vi "Piece_file_Copy.vi"(1 "File Start String":string, 2 "Start to copy file at:":i32, 3 "Source File":path, 4 "Target File":path) -> ()   [LabVIEW 2010]
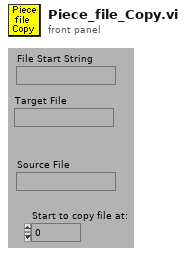
[diagram p1: front panel]
types:
  T1 = enum16{"read/write", "read-only", "write-only", "write-only (truncate)"}
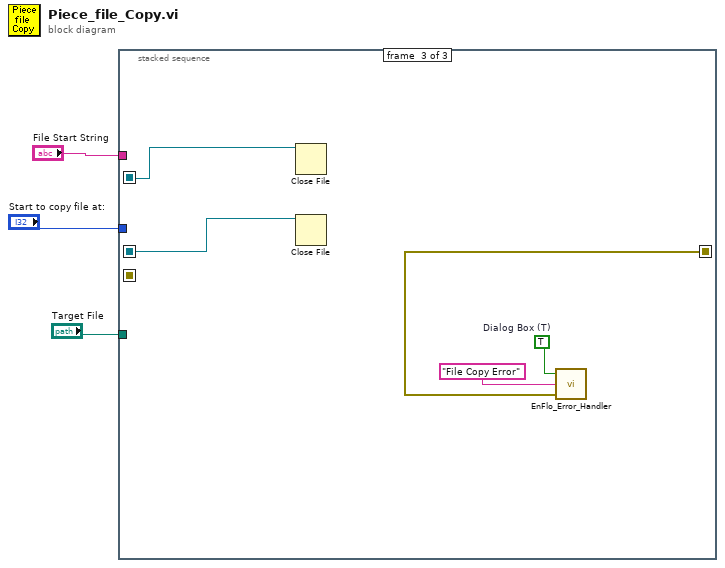
[diagram p0: block diagram]
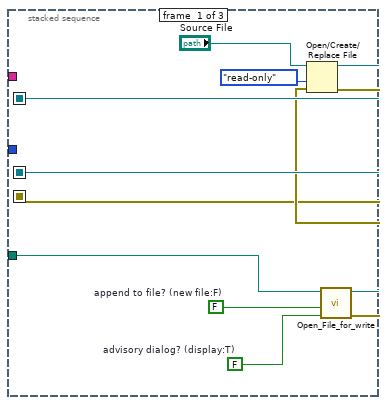
[diagram p2: hidden frame]
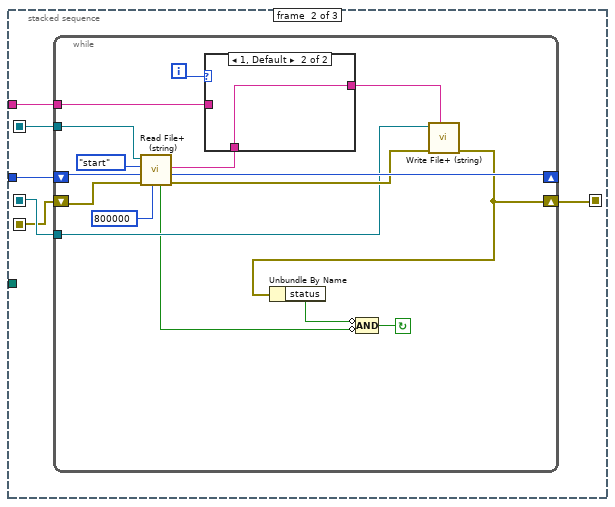
[diagram p3: hidden frame]
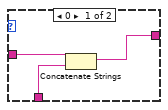
[diagram p4: hidden frame]
diagram:
  n1 = stacked-sequence {
    seq-local: [w9 _ _] -> [_ w18 w43]
    seq-local: [w11 _ _] -> [_ w16 w42]
    seq-local: [w7 _ _] -> [_ w15 _]
    seq-local: [_ w14 _] -> [_ _ w40]
    tunnel: "File Start String" -> [_ w17 _]
    tunnel: "Target File" -> [w6 _ _]
    tunnel: "Start to copy file at:" -> [_ w13 _]
    frame #0 {
      w4 = FALSE  # advisory dialog? (display:T)
      w12 = FALSE  # append to file? (new file:F)
      n2 = call "Open_File_for_write.vi"("advisory dialog? (display:T)"=w4, "append to file? (new file:F)"=w12, "file path"=w6) -> ("error out"=w8:errorcluster, "refnum"=w11:refnum<file>)  [unwired: 7 out]
      n3 = Open/Create/Replace File(file path (use dialog)="Source File", error in=w8, access (0:read/write)=T1."read-only" ("open mode (0)")) -> (refnum out=w9:refnum<file>, error out=w7:errorcluster)  [unwired: 4 out]
    }
    frame #1 {
      n4 = while {
        shift-left: w15 -> [w24]
        shift-right: [w23] -> w14
        tunnel: w16 -> [w26]
        tunnel: w17 -> [w29]
        shift-left: w13 -> [w19]
        shift-right: [w31] -> _
        tunnel: w18 -> [w32]
        i -> [w28]
        stop <- w20 continue-if-true
        n5 = call <vilib>:"Read File+ (string).vi"("count"=800000, "error in (no error)"=w24, "pos offset (bytes:0)"=w19, "pos mode (rel. to current:2)"=enum16{"start", "end", "current"}."start", "refnum"=w32) -> ("error out"=w27:errorcluster, "mark after read (bytes)"=w31:i32, "string"=w30:string, "EOF?"=w21:bool)  [unwired: 3 out]
        n6 = case shown="1, Default" w28 {
          tunnel: w30 -> [w37 w38]
          tunnel: w29 -> [w36 _]
          tunnel: [w35 w38] -> w25
          frame 0 {
            n7 = Concatenate Strings(w36, w37) -> (w35:string)
          }
          frame 1, Default {
          }
        }
        n8 = call <vilib>:"Write File+ (string).vi"("string"=w25, "error in (no error)"=w27, "refnum"=w26) -> ("error out"=w23:errorcluster)  [unwired: 2 in, 4 out]
        n9 = Unbundle By Name(w23) -> ("status"=w22:bool)
        n10 = Compound Arithmetic op=AND(invert w22, invert w21) -> (w20:bool)
      }
    }
    frame #2 {
      w41 = TRUE  # Dialog Box (T)
      n11 = Close File(refnum=w43) -> ()  [unwired: 1 in, 2 out]
      n12 = Close File(refnum=w42) -> ()  [unwired: 1 in, 2 out]
      n13 = call "EnFlo_Error_Handler.vi"("error in (no error)"=w40, "Error Type"="File Copy Error", "Dialog Box (T)"=w41) -> ()  [unwired: 3 out]
    }
  }
